vi "Compile Event Measure 1.0 Data.vi"(8 "error in (no error)":errorcluster, 11 "Device Item Ref in":T3 format="%.0x") -> (0 "error out":errorcluster, 2 "Event Timing Measures":T1[](array[typedef]), 3 "Device Item Ref out":T3 format="%.0x")   [LabVIEW 2017, in "Engine Simulation Toolkit System Explorer.lvlib"]
uses:
  Engine Simulation Toolkit System Explorer.lvlib
  <vilib>/NI Veristand/Custom Device API/Custom Device Item Ref.ctl
  Shared/1.0 Event Timing Measure Engine Data.ctl
  Shared/1.0 Event Timing Measure FIFO Idxs.ctl
  <vilib>/NI Veristand/Custom Device Tools/Custom Device Utility Library/Search Direction.ctl
  Polarity.ctl
  Shared/Constants and GUIDs.vi
  <vilib>/NI Veristand/Custom Device Tools/Custom Device Utility Library/NI VeriStand - Search for Item by GUID.vi
  <vilib>/NI Veristand/Custom Device Tools/Custom Device Utility Library/NI VeriStand - Search for All Items by GUID.vi
  Shared/Engine Simulation Toolkit Shared.lvlib
  <vilib>/NI Veristand/Custom Device Tools/Custom Device Utility Library/Custom Device Utility Library.lvlib
  <vilib>/NI Veristand/Custom Device API/Custom Device API.lvlib
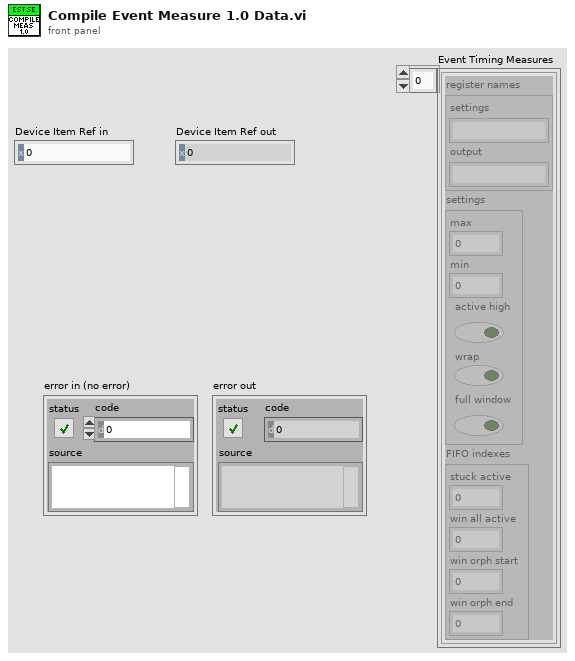
[diagram p1: front panel]
types:
  T1 = typedef "Engine Simulation Toolkit Shared.lvlib/1.0 Event Timing Measure Engine Data.ctl" = cluster{"register names":cluster{"settings":string, "output":string}, "settings":cluster{"max":u16, "min":u16, "active high":bool, "wrap":bool, "full window":bool}, "FIFO indexes":T2}
  T2 = typedef "Engine Simulation Toolkit Shared.lvlib/1.0 Event Timing Measure FIFO Idxs.ctl" = cluster{"stuck active":i32, "win all active":i32, "win orph start":i32, "win orph end":i32}
  T3 = typedef "Custom Device API.lvlib/Custom Device Item Ref.ctl" = u64
  T4 = typedef "Custom Device Utility Library.lvlib/Search Direction.ctl" = enum16{"Down", "Up"}
  T5 = typedef "Engine Simulation Toolkit Shared.lvlib/Channel.ctl" = cluster{"Name":string, "Units":string, "Default":dbl, "Description":string, "Scalable":bool}
  T6 = typedef "Custom Device API.lvlib/Custom Device Item Info.ctl" = cluster{"Name":string, "Is Channel":bool, "GUID":string, "Is Waveform":bool}
  T7 = typedef "Engine Simulation Toolkit System Explorer.lvlib/Event Timing Window.ctl" = cluster{"Name":string, "Min":dbl, "Max":dbl, "Ref":dbl}
  T8 = typedef "Engine Simulation Toolkit System Explorer.lvlib/Event Timing Measurement.ctl" = cluster{"Name":string, "Bitfile name":string, "Window":string, "Polarity":T9}
  T9 = typedef "Engine Simulation Toolkit System Explorer.lvlib/Polarity.ctl" = enum16{"Active low", "Active high"}
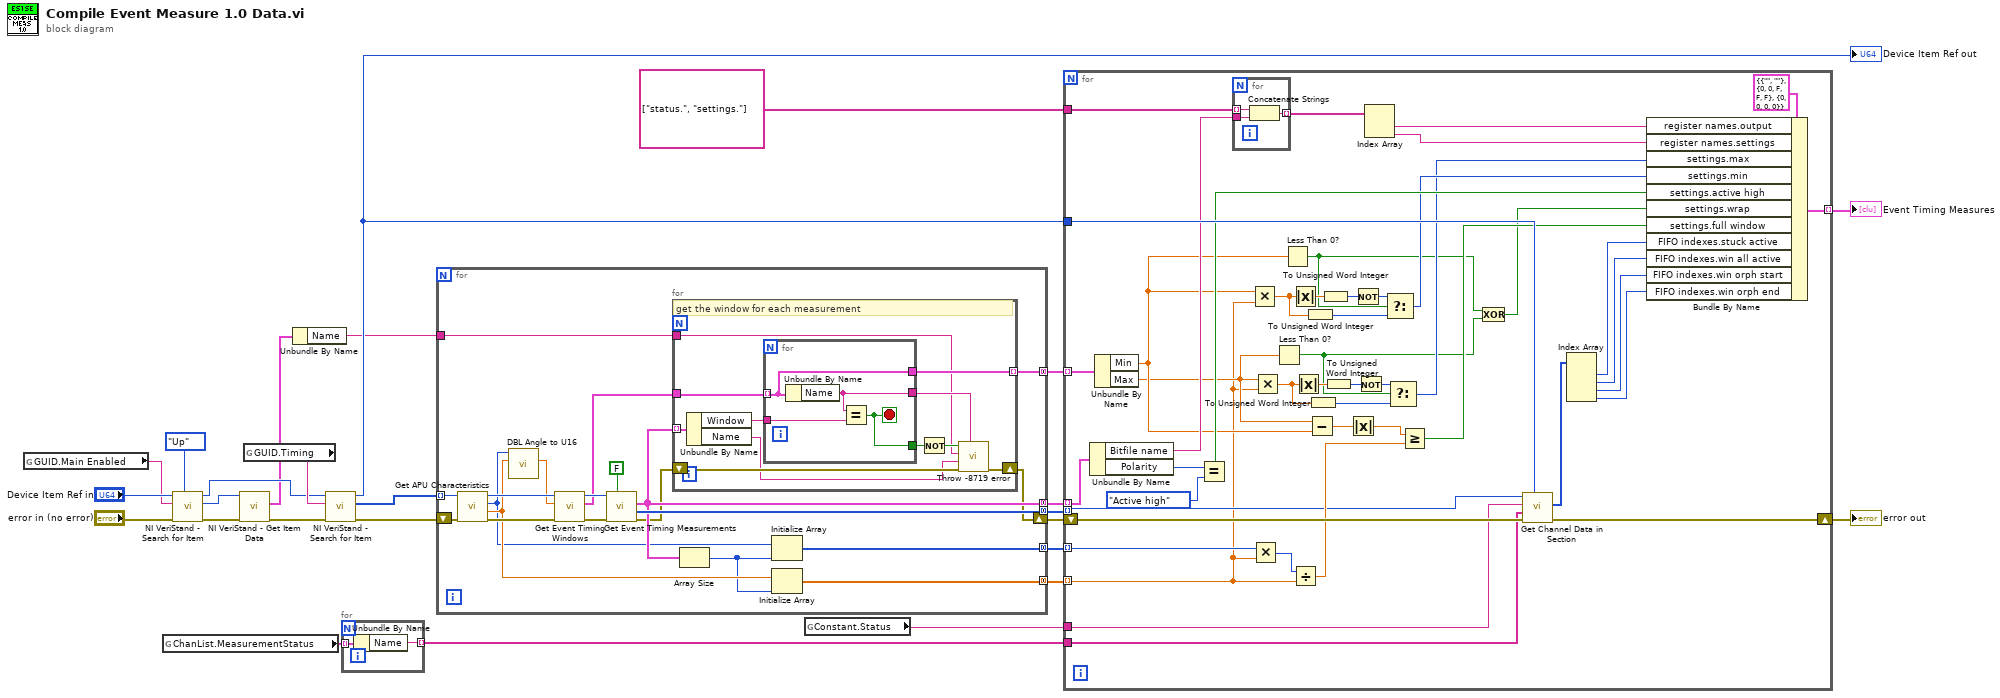
[diagram p0: block diagram]
diagram:
  n1 = global read "Constants and GUIDs.vi" "GUID.Main Enabled"() -> (w7:string)
  n2 = global read "Constants and GUIDs.vi" "ChanList.MeasurementStatus"() -> (w20:T5[])
  n3 = call-poly <vilib>:"NI VeriStand - Search for Item.vi"("Direction (Down)"=Search_Direction."Up", "error in"="error in (no error)", "Item GUID"=w7, "Section Ref in"="Device Item Ref in") -> ("error out"=w9:errorcluster, "Item Ref"=w4:T3, "Section Ref out"=w3:T3)  [unwired: 4 in, 1 out]
  n4 = call <vilib>:"NI VeriStand - Get Item Data.vi"("error in (no error)"=w9, "Item Ref in"=w4) -> ("error out"=w5:errorcluster, "Item Info"=w2:T6)  [unwired: 6 in, 2 out]
  n5 = global read "Constants and GUIDs.vi" "GUID.Timing"() -> (w18:string)
  n6 = Unbundle By Name(w2) -> ("Name"=w1:string)
  n7 = call-poly <vilib>:"NI VeriStand - Search for Item.vi"("error in"=w5, "Item GUID"=w18, "Section Ref in"=w3) -> ("error out"=w25:errorcluster, "Item Refs"=w16:T3[], "Section Ref out"=w21:T3)  [unwired: 5 in, 1 out]
  "Device Item Ref out" <- w21
  n8 = for {
    tunnel: w20 -> [w28] mode=indexing
    tunnel: [w27] -> w19 mode=indexing
    n9 = Unbundle By Name(w28) -> ("Name"=w27:string)
  }
  n10 = for {
    tunnel: w16 -> [w43] mode=indexing
    shift-right: [w31] -> w17
    shift-left: w25 -> [w48]
    tunnel: [w38] -> w15 mode=concatenating
    tunnel: [w47] -> w14 mode=concatenating
    tunnel: [w39] -> w13 mode=concatenating
    tunnel: [w36] -> w12 mode=concatenating
    tunnel: [w33] -> w11 mode=concatenating
    tunnel: w1 -> [w30]
    n11 = call "Get APU Characteristics.vi"("error in (no error)"=w48, "Item Ref in"=w43) -> ("error out"=w44:errorcluster, "angle to u16 scale factor"=w37:dbl, "total angle span (degrees)"=w34:u16, "Item Ref out"=w42:T3)  [unwired: 3 in, 3 out]
    n12 = call "DBL Angle to U16.vi"("angle to u16 scale factor"=w37, "Desired angle (degrees)"=w34) -> ("Actual angle (degrees)"=w41:dbl)  [unwired: 8 in, 1 out]
    n13 = call "Get Event Timing Windows.vi"("error in (no error)"=w44, "Max engine angle"=w41, "Item Ref in"=w42) -> ("error out"=w46:errorcluster, "Windows"=w40:T7[], "Item Ref out"=w45:T3)  [unwired: 6 in]
    n14 = call "Get Event Timing Measurements.vi"("return not-added measurements (T)"=FALSE, "error in (no error)"=w46, "Item Ref in"=w45) -> ("error out"=w32:errorcluster, "measurements refs"=w47:T3[], "measurements"=w38:T8[])  [unwired: 4 in, 2 out]
    n15 = for {
      tunnel: w38 -> [w59] mode=indexing
      tunnel: w40 -> [w58]
      tunnel: [w56] -> w39 mode=indexing
      shift-right: [w52] -> w31
      shift-left: w32 -> [w51]
      tunnel: w30 -> [w49]
      # "get the window for each measurement"
      n16 = Unbundle By Name(w59) -> ("Window"=w57:string, "Name"=w50:string)
      n17 = for {
        tunnel: w58 -> [w62] mode=indexing
        tunnel: w57 -> [w63]
        tunnel: [w62] -> w56
        tunnel: [w61] -> w55
        tunnel: [w60] -> w53
        stop <- w61 stop-if-true
        n18 = Unbundle By Name(w62) -> ("Name"=w60:string)
        n19 = Equal?(x=w60, y=w63) -> (x = y?=w61:bool)
      }
      n20 = Not(x=w55) -> (.not. x?=w54:bool)
      n21 = call "Throw -8719 error.vi"("window name"=w53, "error in (no error)"=w51, "measurement name"=w50, "Custom device name"=w49, "Error"=w54) -> ("error out"=w52:errorcluster)  [unwired: 6 in]
    }
    n22 = Array Size(array=w38) -> (size(s)=w35:i32)
    n23 = Initialize Array(w34, w35) -> (w33:u16[])
    n24 = Initialize Array(w37, w35) -> (w36:dbl[])
  }
  n25 = global read "Constants and GUIDs.vi" "Constant.Status"() -> (w10:string)
  n26 = for {
    shift-right: [w103] -> w23
    shift-left: w17 -> [w106]
    tunnel: string[] ["status.", "settings."] -> [w110]
    tunnel: w19 -> [w104]
    tunnel: [w108] -> w22 mode=indexing
    tunnel: w21 -> [w105]
    tunnel: w15 -> [w94] mode=indexing
    tunnel: w14 -> [w77] mode=indexing
    tunnel: w13 -> [w95] mode=indexing
    tunnel: w12 -> [w69] mode=indexing
    tunnel: w11 -> [w86] mode=indexing
    tunnel: w10 -> [w76]
    n27 = Unbundle By Name(w94) -> ("Bitfile name"=w93:string, "Polarity"=w92:T9)
    n28 = Unbundle By Name(w95) -> ("Min"=w79:dbl, "Max"=w70:dbl)
    n29 = Equal?(x=w92, y=Polarity."Active high") -> (x = y?=w90:bool)
    n30 = for {
      tunnel: w110 -> [w113] mode=indexing
      tunnel: [w112] -> w107 mode=indexing
      tunnel: w93 -> [w111]
      n31 = Concatenate Strings(w113, w111) -> (w112:string)
    }
    n32 = Multiply(x=w79, y=w69) -> (x*y=w80:dbl)
    n33 = Multiply(x=w86, y=w69) -> (x*y=w87:u16)
    n34 = Multiply(x=w70, y=w69) -> (x*y=w71:dbl)
    n35 = Less Than 0?(x=w70) -> (x < 0?=w66:bool)
    n36 = Less Than 0?(x=w79) -> (x < 0?=w65:bool)
    n37 = Absolute Value(x=w80) -> (abs(x)=w82:dbl)
    n38 = Divide(x=w87, y=w69) -> (x/y=w85:dbl)
    n39 = Absolute Value(x=w71) -> (abs(x)=w74:dbl)
    n40 = To Unsigned Word Integer(number=w80) -> (unsigned 16bit integer=w84:u16)
    n41 = Subtract(x=w70, y=w79) -> (x-y=w89:dbl)
    n42 = To Unsigned Word Integer(number=w71) -> (unsigned 16bit integer=w72:u16)
    n43 = To Unsigned Word Integer(number=w82) -> (unsigned 16bit integer=w81:u16)
    n44 = To Unsigned Word Integer(number=w74) -> (unsigned 16bit integer=w75:u16)
    n45 = Absolute Value(x=w89) -> (abs(x)=w68:dbl)
    n46 = Not(x=w81) -> (.not. x?=w83:u16)
    n47 = Not(x=w75) -> (.not. x?=w73:u16)
    n48 = Index Array(array=w107) -> (element #1=w101:string, element #2=w100:string)  [unwired: 2 in]
    n49 = Select(t=w83, s=w65, f=w84) -> (s? t:f=w78:u16)
    n50 = Select(t=w73, s=w66, f=w72) -> (s? t:f=w67:u16)
    n51 = Greater Or Equal?(x=w68, y=w85) -> (x >= y?=w88:bool)
    n52 = Exclusive Or(1:w66, 2:w65) -> (0:w64:bool)
    n53 = call "Get Channel Data in Section.vi"("Custom device ref"=w105, "error in (no error)"=w106, "Channels"=w104, "Section (\"\":none)"=w76, "Item Ref in"=w77) -> ("error out"=w103:errorcluster, "FIFO indexes"=w102:i32[])  [unwired: 2 in, 3 out]
    n54 = Index Array(array=w102) -> (element #1=w99:i32, element #2=w98:i32, element #3=w97:i32, element #4=w96:i32)  [unwired: 4 in]
    n55 = Bundle By Name(cluster=T1 {"register names"={"settings"="", "output"=""}, "settings"={"max"=0, "min"=0, "active high"=FALSE, "wrap"=FALSE, "full window"=FALSE}, "FIFO indexes"={"stuck active"=0, "win all active"=0, "win orph start"=0, "win orph end"=0}} ("1.0.0 Event Timing Measure"), "register names.output"=w101, "register names.settings"=w100, "settings.max"=w67, "settings.min"=w78, "settings.active high"=w90, "settings.wrap"=w64, "settings.full window"=w88, "FIFO indexes.stuck active"=w99, "FIFO indexes.win all active"=w98, "FIFO indexes.win orph start"=w97, "FIFO indexes.win orph end"=w96) -> (w108:T1)
  }
  "error out" <- w23
  "Event Timing Measures" <- w22
